vi "S2DS_GenerateLinePlotArray.vi"(1 "X axis":u16, 2 "Y axis":u16, 3 "Cluster in":T1) -> (0 "Array":T3(array[cluster]))   [LabVIEW 2025]
uses:
  TYPE DEFS/S2DS_PlotInfo.ctl
  TYPE DEFS/S2DS_PlotCluster.ctl
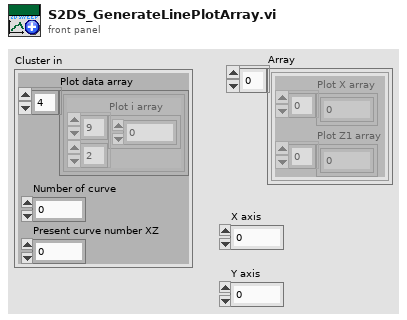
[diagram p1: front panel]
types:
  T1 = typedef "S2DS_PlotInfo.ctl" = cluster{"Plot data array":T2, "Number of curve":i32, "Present curve number XZ":i32}
  T2 = typedef "S2DS_PlotCluster.ctl" = cluster{"Plot i array":dbl[][]}[]
  T3 = cluster{"Plot X array":dbl[], "Plot Z1 array":dbl[]}[]
  T4 = cluster{"Plot i array":dbl[], "Plot i array":dbl[]}
  T5 = cluster{"Plot i array":dbl[], "Plot i array":dbl[]}[]
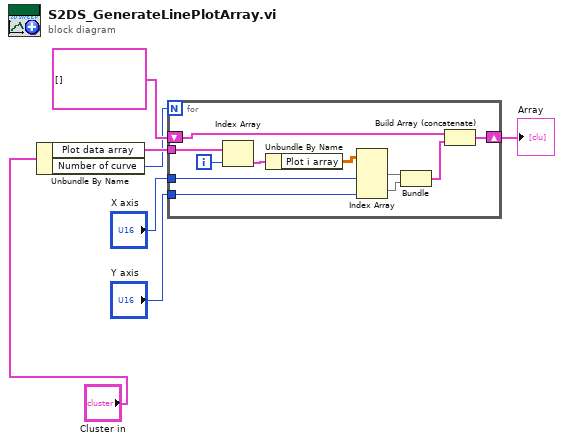
[diagram p0: block diagram]
diagram:
  n1 = Unbundle By Name("Cluster in") -> ("Plot data array"=w3:T2, "Number of curve"=w2:i32)
  n2 = for {
    N: w2 -> [_]
    tunnel: w3 -> [w18]
    shift-right: [w16] -> w5
    shift-left: T3 [] -> [w15]
    tunnel: "X axis" -> [w11]
    tunnel: "Y axis" -> [w10]
    i -> [w17]
    n3 = Index Array(array=w18, index=w17) -> (element=w13:cluster{"Plot i array":dbl[][]})
    n4 = Unbundle By Name(w13) -> ("Plot i array"=w12:dbl[][])
    n5 = Index Array(array=w12, index (col) #1=w11, index (col) #2=w10) -> (element #1=w9:dbl[], element #2=w8:dbl[])  [unwired: 2 in]
    n6 = Bundle("Plot i array"=w9, "Plot i array"=w8) -> (w14:T4)  [unwired: 1 in]
    n7 = Build Array (concatenate)(w15, w14) -> (w16:T5)
  }
  "Array" <- w5
